vi "SubVI_transdutor_laser.vi"(0 "Numeric Control 2":u8, 1 "I2C Ref Out in":T1, 2 "Array in":u16[](array[numeric]), 3 "array in":dbl[](array[numeric]), 4 "array 3":dbl[](array[numeric]), 5 "mean in":dbl, 6 "Numeric Control 3":i32, 7 "error in (no error)":errorcluster, 8 "io_timeout":u16, 9 "Numeric Control":i32, 10 "y 2":u16, 12 "y":u16) -> (16 "Range":u16, 18 "Boolean":bool, 20 "I2C Ref Out out":T1, 21 "did_timeout":bool, 22 "Numeric Control 4":u32, 23 "Array out":u16[](array[numeric]), 24 "array out":dbl[](array[numeric]), 25 "mean out":dbl, 27 "error out":errorcluster)   [LabVIEW 2017]
uses:
  <vilib>/myRIO/Instrument Drivers/Onboard IO/I2C/typedefs/I2C Reference.ctl
  <vilib>/myRIO/Common/Instrument Driver Framework/Utilities/typedefs/myRIO Generic Hardware Reference.ctl
  <vilib>/myRIO/Common/Instrument Driver Framework/Utilities/typedefs/Hardware Version Enum.ctl
  <vilib>/myRIO/Common/Instrument Driver Framework/Utilities/typedefs/myRIO v1.0 Reference.ctl
  <vilib>/myRIO/Common/Instrument Driver Framework/Utilities/typedefs/Generic FPGA Reference.ctl
  <vilib>/myRIO/Common/Instrument Driver Framework/myRIO v1.0/I2C/typedefs/I2C Channels Enum.ctl
  <vilib>/myRIO/Instrument Drivers/Onboard IO/I2C/typedefs/I2C Configuration.ctl
  <vilib>/myRIO/Instrument Drivers/Onboard IO/I2C/typedefs/I2C Transfer Rate.ctl
  <vilib>/Analysis/baseanly.llb/Mean (DBL).vi
  <vilib>/Analysis/NI_AALBase.lvlib
  <vilib>/myRIO/Instrument Drivers/Onboard IO/I2C/I2C.lvlib
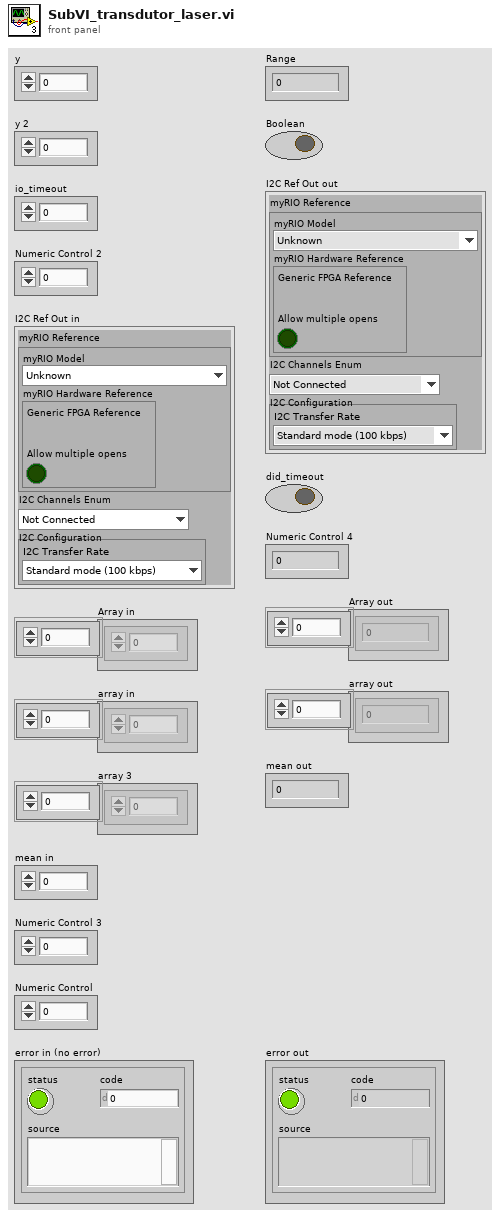
[diagram p1: front panel]
types:
  T1 = typedef "I2C.lvlib/I2C Reference.ctl" = cluster{"myRIO Reference":T2, "I2C Channels Enum":T6, "I2C Configuration":T7}
  T2 = typedef "myRIO Generic Hardware Reference.ctl" = cluster{"myRIO Model":T3, "myRIO Hardware Reference":T4}
  T3 = typedef "Hardware Version Enum.ctl" = enum16{"Unknown", "myRIO-1900", "myRIO-1950", "roboRIO", "NI ELVIS RIO CM"}
  T4 = typedef "myRIO v1.0 Reference.ctl" = cluster{"Generic FPGA Reference":T5, "Allow multiple opens":bool}
  T5 = typedef "Generic FPGA Reference.ctl" = refnum<k20>
  T6 = typedef "I2C Channels Enum.ctl" = enum16{"Not Connected", "A/I2C", "B/I2C", "I2C/I2C"}
  T7 = typedef "I2C.lvlib/I2C Configuration.ctl" = cluster{"I2C Transfer Rate":T8}
  T8 = typedef "I2C.lvlib/I2C Transfer Rate.ctl" = enum16{"Standard mode (100 kbps)", "Fast mode (400 kbps)"}
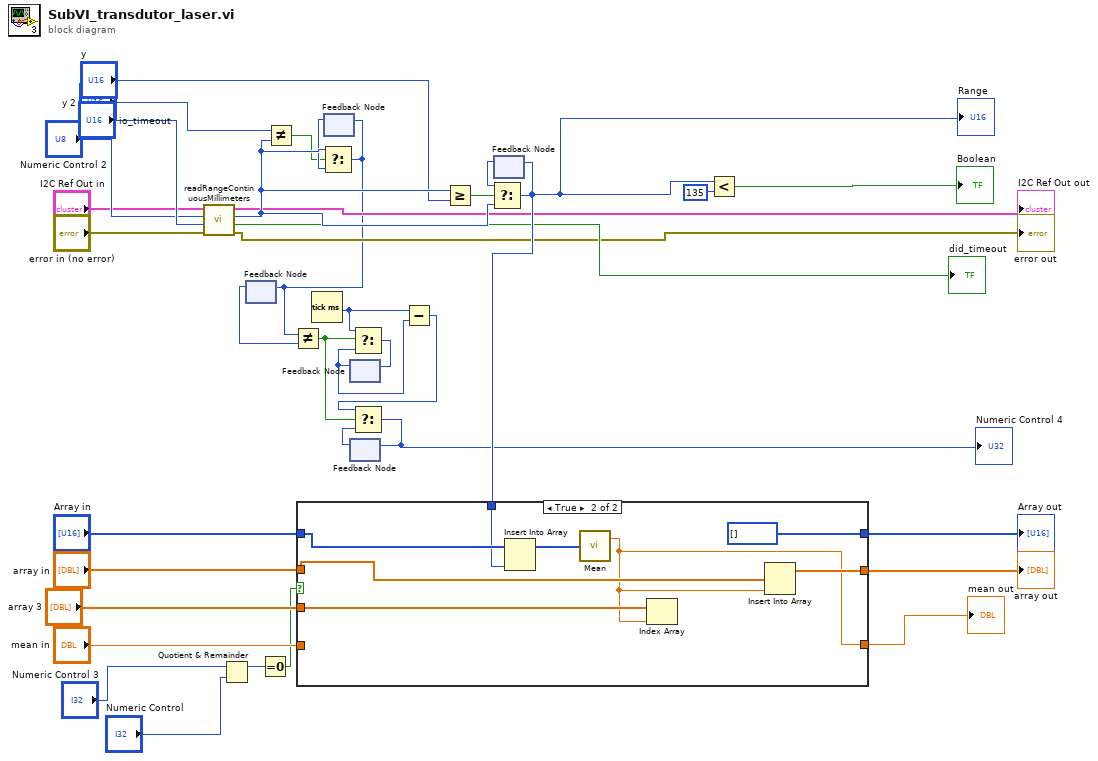
[diagram p0: block diagram]
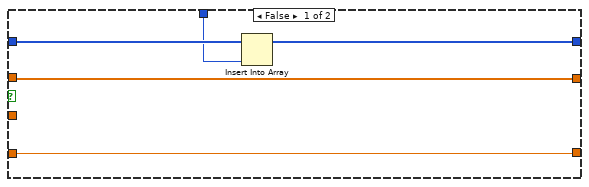
[diagram p2: hidden frame]
diagram:
  n1 = call "readRangeContinuousMillimeters.vi"("error in"="error in (no error)", "io_timeout"="io_timeout", "Slave Address(7 bit)"="Numeric Control 2", "I2C Ref In"="I2C Ref Out in") -> ("error out"=→"error out":errorcluster, "did_timeout"=→"did_timeout":bool, "Range"=w26:u16, "I2C Ref Out"=→"I2C Ref Out out":T1)  [unwired: 4 in]
  n2 = Quotient & Remainder(x="Numeric Control 3", y="Numeric Control") -> (x-y*floor(x/y)=w16:i32)  [unwired: 1 out]
  n3 = feedback #1() -> (w3:u16)  [unwired: 1 in]
  n4 = Equal To 0?(x=w16) -> (x = 0?=w17:bool)
  n5 = Not Equal?(x="y 2", y=w26) -> (x != y?=w1:bool)
  n6 = Tick Count (ms)() -> (millisecond timer value=w5:u32)
  n7 = feedback #2() -> (w2:u16)  [unwired: 1 in]
  n8 = Select(t=w26, s=w1, f=w2) -> (s? t:f=w11:u16)
  n9 = feedback-in #1(w11) -> ()
  n10 = Not Equal?(x=w11, y=w3) -> (x != y?=w7:bool)
  n11 = feedback-in #2(w11) -> ()
  n12 = feedback #3() -> (w6:u32)  [unwired: 1 in]
  n13 = feedback #4() -> (w8:u32)  [unwired: 1 in]
  n14 = Select(t=w5, s=w7, f=w6) -> (s? t:f=w4:u32)
  n15 = feedback-in #3(w4) -> ()
  n16 = Subtract(x=w5, y=w6) -> (x-y=w9:u32)
  n17 = Select(t=w9, s=w7, f=w8) -> (s? t:f=w10:u32)
  "Numeric Control 4" <- w10
  n18 = feedback-in #4(w10) -> ()
  n19 = Greater Or Equal?(x=w26, y="y") -> (x >= y?=w13:bool)
  n20 = feedback #5() -> (w15:u16)  [unwired: 1 in]
  n21 = Select(t=w15, s=w13, f=w26) -> (s? t:f=w30:u16)
  "Range" <- w30
  n22 = case shown="True" w17 {
    tunnel: "Array in" -> [w42 w49]
    tunnel: w30 -> [w41 w48]
    tunnel: [w40 u16[] []] -> w19
    tunnel: "array 3" -> [_ w46]
    tunnel: "array in" -> [w39 w45]
    tunnel: [w39 w44] -> w35
    tunnel: [w38 w43] -> w36
    tunnel: "mean in" -> [w38 _]
    frame False {
      n23 = Insert Into Array(array=w42, new element=w41) -> (w40:u16[])  [unwired: 1 in]
    }
    frame True {
      n24 = Insert Into Array(array=w49, new element=w48) -> (w47:u16[])  [unwired: 1 in]
      n25 = call-poly <vilib>:"Mean.vi"("X"=w47) -> ("mean"=w43:dbl)  [unwired: 1 out]
      n26 = Index Array(array=w46, index=w43) -> ()  [unwired: 1 out]
      n27 = Insert Into Array(array=w45, new element=w43) -> (w44:dbl[])  [unwired: 1 in]
    }
  }
  "mean out" <- w36
  "array out" <- w35
  "Array out" <- w19
  n28 = feedback-in #5(w30) -> ()
  n29 = Less?(x=w30, y=u16 135) -> (x < y?=→"Boolean":bool)
